vi "PumpAcid.vi"(1 "relay session in":T1={"VISA resource out"="COM12", "error out"={"status"=FALSE, "code"=0, "source"=""}}) -> (0 "relay session out":T1={"VISA resource out"="COM12", "error out"={"status"=FALSE, "code"=0, "source"=""}})   [LabVIEW 2010]
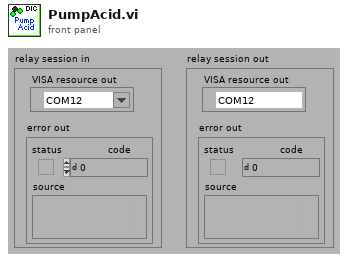
[diagram p1: front panel]
types:
  T1 = cluster{"VISA resource out":refnum<visa-resource-name>, "error out":errorcluster}
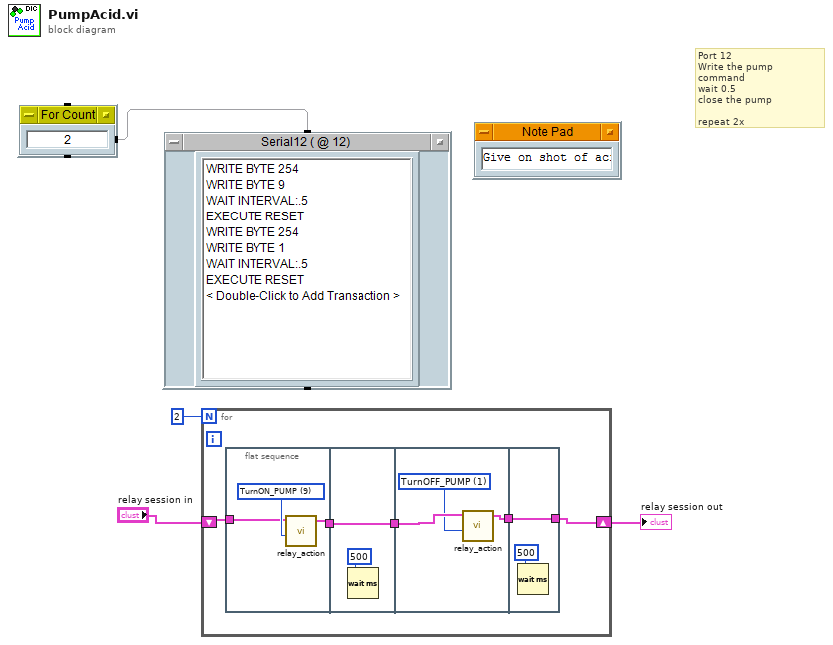
[diagram p0: block diagram]
diagram:
  # "Port 12\nWrite the pump command \nwait 0.5 \nclose the pump\n\nrepeat 2x"
  n1 = for {
    N: 2 -> [_]
    shift-right: [w4] -> w1
    shift-left: "relay session in" -> [w5]
    n2 = flat-sequence {
      tunnel: [w10] -> w7
      tunnel: w5 -> [w9]
      tunnel: [w12] -> w8
      tunnel: w7 -> [w12]
      tunnel: w8 -> [w16]
      tunnel: [w14] -> w6
      tunnel: [w18] -> w4
      tunnel: w6 -> [w18]
      frame #0 {
        w11 = u8 9 items=["TurnON_1"=8, "TurnON_PUMP"=9, "TurnON_3"=10, "TurnON_4"=11, "TurnOFF_1"=0, "TurnOFF_PUMP"=1, "TurnOFF_3"=2, "TurnOFF_4"=3, "OpenAll"=30, "CloseAllRelay"=29] ("Action")
        n3 = call "relay_action.vi"("relay session in"=w9, "Action"=w11) -> ("relay session out"=w10:T1)  [unwired: 6 in]
      }
      frame #1 {
        n4 = Wait (ms)(milliseconds to wait=500) -> ()  [unwired: 1 out]
      }
      frame #2 {
        w15 = u8 1 items=["TurnON_1"=8, "TurnON_PUMP"=9, "TurnON_3"=10, "TurnON_4"=11, "TurnOFF_1"=0, "TurnOFF_PUMP"=1, "TurnOFF_3"=2, "TurnOFF_4"=3, "OpenAll"=30, "CloseAllRelay"=29] ("Action 2")
        n5 = call "relay_action.vi"("relay session in"=w16, "Action"=w15) -> ("relay session out"=w14:T1)  [unwired: 6 in]
      }
      frame #3 {
        n6 = Wait (ms)(milliseconds to wait=500) -> ()  [unwired: 1 out]
      }
    }
  }
  "relay session out" <- w1
